vi "demandsView.vi"(10 "UserEvents in":refnum<class "UserEvents.lvclass">) -> ()   [LabVIEW 2015, in "M1M3SSSTViews.lvlib"]
uses:
  M1M3SSSTViews.lvlib
  UserEvents/UserEvents.lvclass
  CommandFactory/CommandFactory.lvclass
  UserEvents/UserEvents.lvclass/UserEvents.ctl
  Typedefs/StateSelector.ctl
  Typedefs/CommandSelector.ctl
  Typedefs/M1M3SSSTypedefs.lvlib
  ConfigurationTestParameters/ConfigurationTestParameters.lvclass
panel:
  in  "stopTestIsTrue":bool
  in  "startTestIsTrue":bool
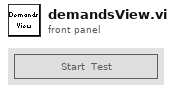
[diagram p1: front panel]
types:
  T1 = enum8{"Enabled", "Disabled", "Disabled and Grayed Out"}
  T2 = typedef "M1M3SSSTypedefs.lvlib/PubDataEvents.ctl" = cluster{"State":refnum<user-event>, "ErrorCode":refnum<user-event>, "OutputData":refnum<user-event>, "InputData":refnum<user-event>, "ControllerData":refnum<user-event>, "TestStatus":refnum<user-event>, "LogPath":refnum<user-event>, "StiffnessData":refnum<user-event>, "PreconditioningCycle":refnum<user-event>}
  T3 = typedef "M1M3SSSTypedefs.lvlib/SubDataEvents.ctl" = cluster{"Command":refnum<user-event>}
  T4 = cluster{"Event Registration Refnum":refnum<event-registration>}
  T5 = typedef "M1M3SSSTypedefs.lvlib/StateSelector.ctl" = enum16{"FaultState", "OffState", "RampingUpPressurePState", "RampingUpPressureSTState", "StandbyState", "StoppedState", "WaitingForSettledPState", "WaitingForSettledSTState"}
  T6 = typedef "M1M3SSSTypedefs.lvlib/CommandSelector.ctl" = enum16{"ClearError", "Exit", "StandBy", "Start", "StartTest", "StopTest", "Update"}
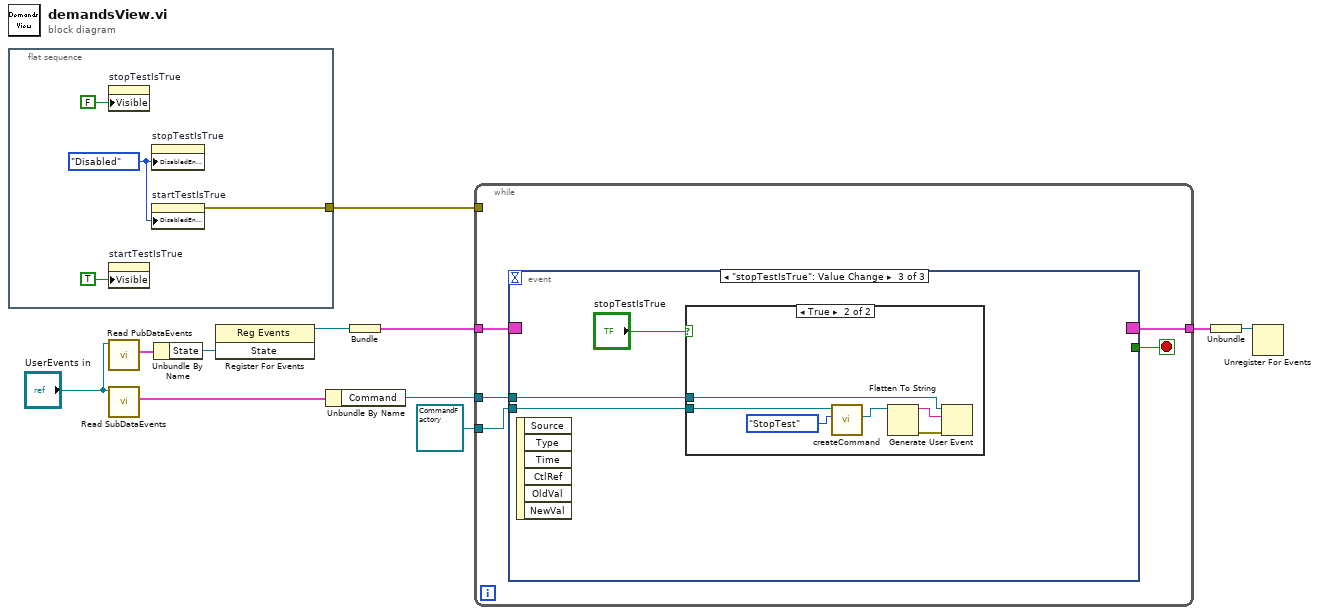
[diagram p0: block diagram]
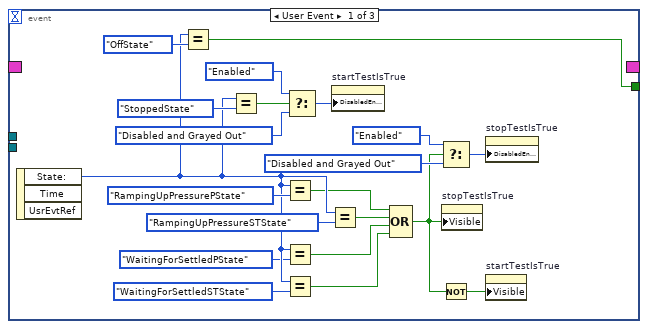
[diagram p2: hidden frame]
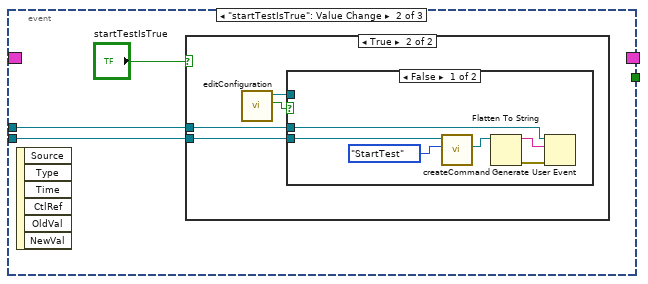
[diagram p3: hidden frame]
diagram:
  n1 = flat-sequence {
    tunnel: [w12] -> w1
    frame #0 {
      w15 = T1."Disabled" ("Disabled")
      n2 = property on="stopTestIsTrue" class="Bool"("Visible"=FALSE) -> ()  [unwired: 2 in, 2 out]
      n3 = property on="startTestIsTrue" class="Bool"("Visible"=TRUE) -> ()  [unwired: 2 in, 2 out]
      n4 = property on="stopTestIsTrue" class="Bool"("DisabledEnum"=w15) -> ()  [unwired: 2 in, 2 out]
      n5 = property on="startTestIsTrue" class="Bool"("DisabledEnum"=w15) -> (error out=w12:errorcluster)  [unwired: 2 in, 1 out]
    }
  }
  n6 = call "Read PubDataEvents.vi"("UserEvents in"="UserEvents in") -> ("PubDataEvents"=w8:T2)  [unwired: 9 in, 1 out]
  n7 = call "Read SubDataEvents.vi"("UserEvents in"="UserEvents in") -> ("SubDataEvents"=w9:T3)  [unwired: 9 in, 1 out]
  n8 = Unbundle By Name(w8) -> ("State"=w10:refnum<user-event>)
  n9 = register-events(w10) -> (reference out=w11:refnum<event-registration>)  [unwired: 2 in, 1 out]
  n10 = Unbundle By Name(w9) -> ("Command"=w6:refnum<user-event>)
  n11 = Bundle("Event Registration Refnum"=w11) -> (w7:T4)  [unwired: 1 in]
  n12 = while {
    tunnel: w7 -> [w20]
    tunnel: w6 -> [w19]
    tunnel: [w18] -> w5
    tunnel: refnum<class "CommandFactory.lvclass"> refnum ("CommandFactory.lvclass") -> [w16]
    tunnel: w1 -> [_]
    stop <- w17 stop-if-true
    n13 = event shown="[2] \"stopTestIsTrue\": Value Change" {
      selector: w20 -> [_ _ _]
      dyn-events: [_ _ _] -> w18
      timeout: _ -> [_ _ _]
      tunnel: w19 -> [_ w42 w57]
      tunnel: [w40 _ _] -> w17
      tunnel: w16 -> [_ w43 w56]
      event User Event {
        n14 = event-data() -> ("State:"=w29:T5)  [unwired: 1 in, 2 out]
        n15 = Equal?(x=w29, y=StateSelector."OffState") -> (x = y?=w40:bool)
        n16 = Equal?(x=w29, y=StateSelector."StoppedState" ("State:")) -> (x = y?=w33:bool)
        n17 = Equal?(x=w29, y=StateSelector."RampingUpPressurePState" ("State:")) -> (x = y?=w25:bool)
        n18 = Equal?(x=w29, y=StateSelector."WaitingForSettledPState" ("State:")) -> (x = y?=w23:bool)
        n19 = Equal?(x=w29, y=StateSelector."WaitingForSettledSTState" ("State:")) -> (x = y?=w22:bool)
        n20 = Select(t=T1."Enabled" ("Disabled"), s=w33, f=T1."Disabled and Grayed Out" ("Disabled")) -> (s? t:f=w32:T1)
        n21 = Equal?(x=w29, y=StateSelector."RampingUpPressureSTState" ("State:")) -> (x = y?=w24:bool)
        n22 = property on="startTestIsTrue" class="Bool"("DisabledEnum"=w32) -> ()  [unwired: 2 in, 2 out]
        n23 = Compound Arithmetic op=OR(w25, w24, w23, w22) -> (w21:bool)
        n24 = Select(t=T1."Enabled" ("Disabled"), s=w21, f=T1."Disabled and Grayed Out" ("Disabled")) -> (s? t:f=w36:T1)
        n25 = Not(x=w21) -> (.not. x?=w34:bool)
        n26 = property on="stopTestIsTrue" class="Bool"("Visible"=w21) -> ()  [unwired: 2 in, 2 out]
        n27 = property on="stopTestIsTrue" class="Bool"("DisabledEnum"=w36) -> ()  [unwired: 2 in, 2 out]
        n28 = property on="startTestIsTrue" class="Bool"("Visible"=w34) -> ()  [unwired: 2 in, 2 out]
      }
      event "startTestIsTrue": Value Change {
        n29 = event-data() -> ()  [unwired: 1 in, 6 out]
        n30 = case shown="True" "startTestIsTrue" {
          tunnel: w43 -> [_ w48]
          tunnel: w42 -> [_ w47]
          frame False {
          }
          frame True {
            n31 = call "editConfiguration.vi"() -> ("cancelIsTrue out"=w45:bool, "ConfigurationThisComponent out"=w46:refnum<class "ConfigurationTestParameters.lvclass">)  [unwired: 9 in, 1 out]
            n32 = case shown="False" w45 {
              tunnel: w48 -> [w54 _]
              tunnel: w47 -> [w51 _]
              tunnel: w46 -> [_ _]
              frame False {
                n33 = call-dynamic "createCommand.vi"("Command"=CommandSelector."StartTest", "CommandFactory in"=w54) -> ("command"=w50:refnum<class "Command.lvclass">)  [unwired: 7 in, 2 out]
                n34 = Flatten To String(anything=w50) -> (data string=w52:string, error out=w53:errorcluster)  [unwired: 3 in, 1 out]
                n35 = Generate User Event(user event=w51, event data cluster=w52, error in=w53) -> ()  [unwired: 1 in, 2 out]
              }
              frame True {
              }
            }
          }
        }
      }
      event "stopTestIsTrue": Value Change {
        n36 = event-data() -> ()  [unwired: 1 in, 6 out]
        n37 = case shown="True" "stopTestIsTrue" {
          tunnel: w56 -> [_ w63]
          tunnel: w57 -> [_ w60]
          frame False {
          }
          frame True {
            n38 = call-dynamic "createCommand.vi"("Command"=CommandSelector."StopTest", "CommandFactory in"=w63) -> ("command"=w59:refnum<class "Command.lvclass">)  [unwired: 7 in, 2 out]
            n39 = Flatten To String(anything=w59) -> (data string=w61:string, error out=w62:errorcluster)  [unwired: 3 in, 1 out]
            n40 = Generate User Event(user event=w60, event data cluster=w61, error in=w62) -> ()  [unwired: 1 in, 2 out]
          }
        }
      }
    }
  }
  n41 = Unbundle(w5) -> ("Event Registration Refnum"=w4:refnum<event-registration>)
  n42 = Unregister For Events(event registration refnum=w4) -> ()  [unwired: 1 in, 1 out]
